vi "Write message.vi"(8 "error in (no error)":errorcluster, 10 "message":T1, 11 "message_text in":refnum<class "message_text.lvclass">) -> (0 "error out":errorcluster, 3 "message_text out":refnum<class "message_text.lvclass">)   [LabVIEW 2020, in "message_text.lvclass"]
uses:
  message_text.lvclass
  message.ctl
  message_text.lvclass/message_text.ctl
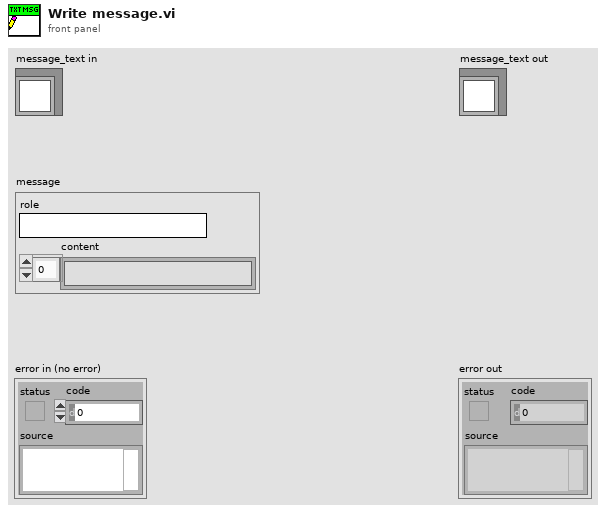
[diagram p1: front panel]
types:
  T1 = typedef "message_text.lvclass/message.ctl" = cluster{"role":string, "content":string[]}
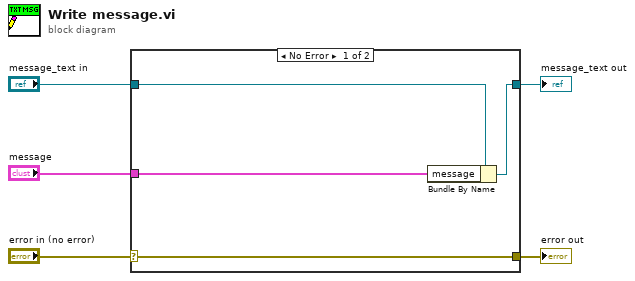
[diagram p0: block diagram]
diagram:
  n1 = case shown="No Error" "error in (no error)" {
    selector: "error in (no error)" -> [w9 w10]
    tunnel: [w9 w10] -> w4
    tunnel: [w7 w11] -> w2
    tunnel: "message_text in" -> [w8 w11]
    tunnel: "message" -> [w6 _]
    frame No Error {
      n2 = Bundle By Name(cluster=w8, "message"=w6) -> (w7:refnum<class "message_text.lvclass">)
    }
    frame Error {
    }
  }
  "error out" <- w4
  "message_text out" <- w2
